vi "Initialize Work.vi"(6 "Controller name":string, 8 "error in (no error)":errorcluster, 9 "Update period":dbl, 11 "Measure Object in":refnum<class "Worker Actor.lvclass">) -> (0 "error out":errorcluster, 3 "Measure Object out":refnum<class "Worker Actor.lvclass">)   [LabVIEW 2021, in "Worker Actor.lvclass"]
uses:
  Worker Actor.lvclass
  Worker Actor.lvclass/Worker Actor.ctl
  Template Module Messages/Result Reply Msg/Result Reply Msg.lvclass
  Controllers/Process Controller Messages/Stop Measurements Msg/Stop Measurements Msg.lvclass
  NHMFL_Core/Libraries/Instruments/Instrument Driver/Worker State.ctl
  NHMFL_Core/Libraries/Instruments/Results/Acquired Result/Acquired Result.lvclass
  NHMFL_Core/Libraries/File/Metadata/Metadata.lvclass
  Publish-Subscribe/Context.ctl
  Publish-Subscribe/Interfaces/Subscriber Messages/Information Msg/Information Msg.lvclass
  <vilib>/ActorFramework/Actor/Actor.lvclass
  C:/GitHub/LabActor/Template Module/Template Module.lvclass
  C:/Program Files/National Instruments/LabVIEW 2021/vi.lib/ActorFramework/Actor/Actor.lvclass
  C:/GitHub/LabActor/Worker/Worker Actor/Worker Actor.lvclass
  C:/GitHub/LabActor/Worker/Woker Interface/Worker.lvclass
  C:/GitHub/NHMFL_Core/Libraries/Instruments/Results/Acquired Result/Acquired Result.lvclass
  C:/GitHub/LabActor/Publish-Subscribe/Interfaces/Information/Information.lvclass
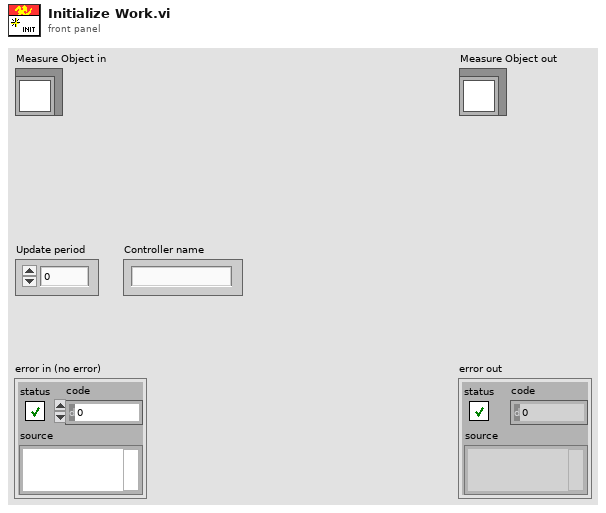
[diagram p1: front panel]
types:
  T1 = typedef "Worker State.ctl" = enum16{"Idle", "Starting", "Working", "Stopping"}
  T2 = typedef "Context.ctl" = cluster{"Topic":string, "Source":string}
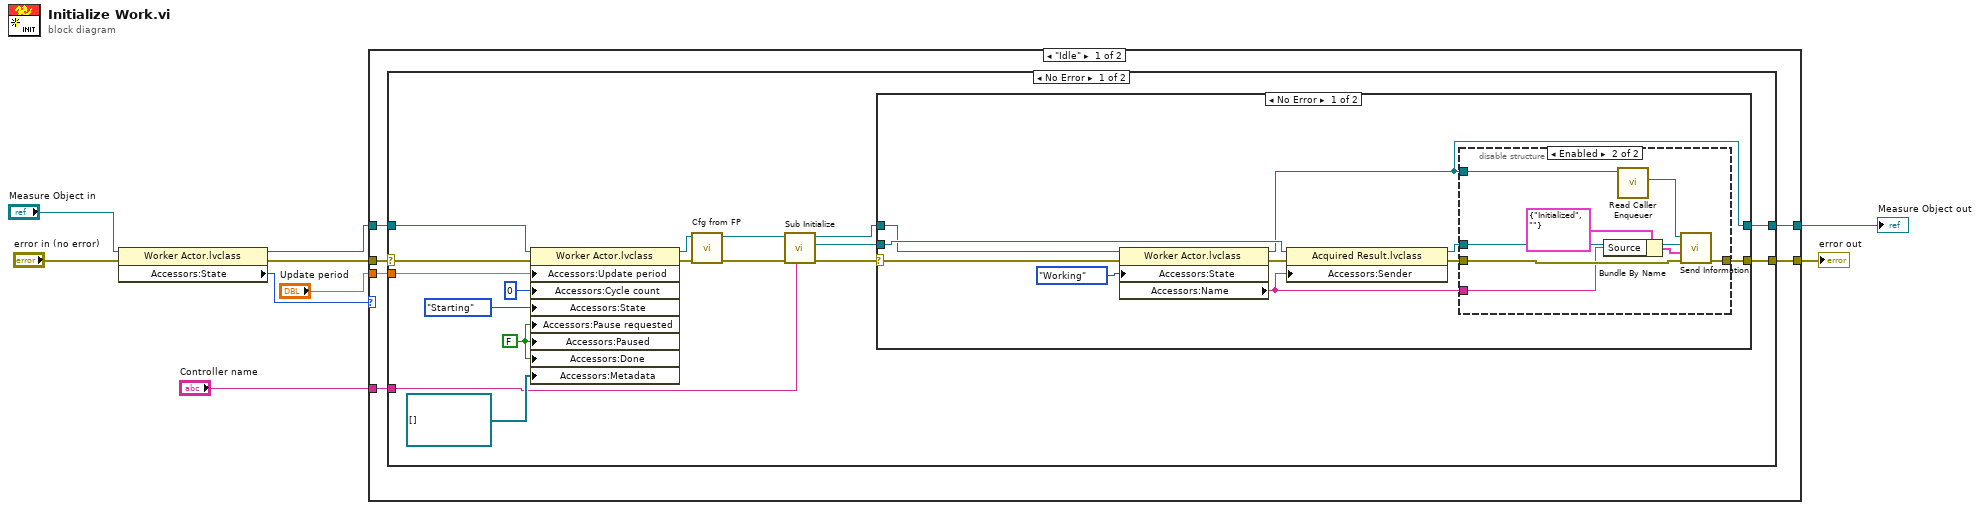
[diagram p0: block diagram]
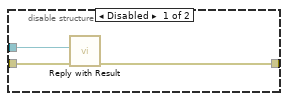
[diagram p2: hidden frame]
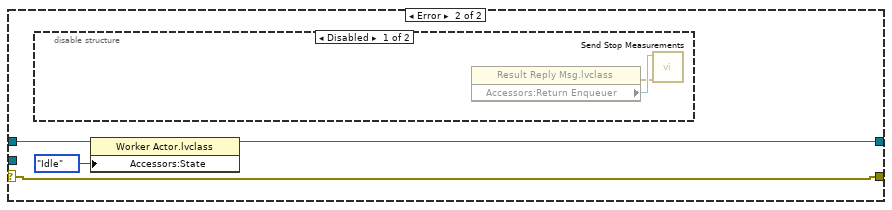
[diagram p3: hidden frame]
diagram:
  n1 = property class="Worker Actor.lvclass"(reference="Measure Object in", error in="error in (no error)") -> (reference out=w5:refnum<class "Worker Actor.lvclass">, error out=w3:errorcluster, "Accessors:State"=w2:T1)
  n2 = case shown="\"Idle\"" w2 {
    tunnel: [w15 w62] -> w9
    tunnel: [w14 w63] -> w8
    tunnel: "Update period" -> [w13 _]
    tunnel: w5 -> [w12 w63]
    tunnel: w3 -> [w11 w62]
    tunnel: "Controller name" -> [w10 _]
    frame "Idle" {
      n3 = case shown="No Error" w11 {
        selector: w11 -> [w26 w61]
        tunnel: [w32 w61] -> w15
        tunnel: [w23 w60] -> w14
        tunnel: w12 -> [w31 w60]
        tunnel: w13 -> [w22 _]
        tunnel: w10 -> [w16 _]
        frame No Error {
          w18 = FALSE ("Pause requested")
          n4 = property class="Worker Actor.lvclass"(reference=w31, error in=w26, "Accessors:Update period"=w22, "Accessors:Cycle count"=0 ("Cycle count"), "Accessors:State"=Worker_State."Starting" ("State"), "Accessors:Pause requested"=w18, "Accessors:Paused"=w18, "Accessors:Done"=w18, "Accessors:Metadata"=refnum<class "Metadata.lvclass">[] [] ("Metadata")) -> (reference out=w27:refnum<class "Worker Actor.lvclass">, error out=w25:errorcluster)
          n5 = call-dynamic "Cfg from FP.vi"("error in (no error)"=w25, "Measure Object in"=w27) -> ("error out"=w28:errorcluster, "Measure Object out"=w30:refnum<class "Worker Actor.lvclass">)  [unwired: 8 in]
          n6 = call-dynamic "Sub Initialize.vi"("Controller name"=w16, "error in (no error)"=w28, "Measure Object in"=w30) -> ("error out"=w21:errorcluster, "Initialize Result"=w29:refnum<class "Acquired Result.lvclass">, "Measure Object out"=w24:refnum<class "Worker Actor.lvclass">)  [unwired: 6 in]
          n7 = case shown="No Error" w21 {
            selector: w21 -> [w36 w56]
            tunnel: [w42 w56] -> w32
            tunnel: w29 -> [w39 _]
            tunnel: w24 -> [w38 w57]
            tunnel: [w34 w55] -> w23
            frame No Error {
              n8 = property class="Worker Actor.lvclass"(reference=w38, error in=w36, "Accessors:State"=Worker_State."Working" ("State")) -> (reference out=w34:refnum<class "Worker Actor.lvclass">, error out=w37:errorcluster, "Accessors:Name"=w33:string)
              n9 = property class="Acquired Result.lvclass"(reference=w39, error in=w37, "Accessors:Sender"=w33) -> (reference out=w40:refnum<class "Acquired Result.lvclass">, error out=w41:errorcluster)
              n10 = disable-structure shown="Enabled" {
                disable-tunnel: [w45 w50] -> w42
                disable-tunnel: w41 -> [w44 w49]
                disable-tunnel: w40 -> [w43 w47]
                disable-tunnel: w34 -> [_ w48]
                disable-tunnel: w33 -> [_ w46]
                frame Disabled {
                  n11 = call-dynamic "Reply with Result.vi"("error in (no error)"=w44, "Result"=w43) -> ("error out"=w45:errorcluster)  [unwired: 8 in, 1 out]
                }
                frame Enabled {
                  n12 = Bundle By Name(cluster=T2 {"Topic"="Initialized", "Source"=""} ("Context"), "Source"=w46) -> (w51:T2)
                  n13 = call <vilib>:"Read Caller Enqueuer.vi"("Actor"=w48) -> ("Caller Enqueuer"=w52:refnum<class "Message Enqueuer.lvclass">)  [unwired: 10 in]
                  n14 = call "Send Information.vi"("error in (no error)"=w49, "Context"=w51, "Information"=w47, "Message Enqueuer"=w52) -> ("error out"=w50:errorcluster)  [unwired: 6 in, 1 out]
                }
              }
            }
            frame Error {
              n15 = disable-structure shown="Disabled" {
                frame Disabled {
                  n16 = property class="Result Reply Msg.lvclass"() -> (error out=w58:errorcluster, "Accessors:Return Enqueuer"=w59:refnum<class "Message Enqueuer.lvclass">)  [unwired: 2 in, 1 out]
                  n17 = call "Send Stop Measurements.vi"("error in (no error)"=w58, "Message Enqueuer"=w59) -> ()  [unwired: 8 in, 2 out]
                }
                frame Enabled {
                }
              }
              n18 = property class="Worker Actor.lvclass"(reference=w57, "Accessors:State"=Worker_State."Idle" ("State")) -> (reference out=w55:refnum<class "Worker Actor.lvclass">)  [unwired: 1 in, 1 out]
            }
          }
        }
        frame Error {
        }
      }
    }
    frame "Working", Default {
    }
  }
  "error out" <- w9
  "Measure Object out" <- w8
